vi "RT_Coriolis_Moment_in_DLR_Navigation_Reference_System(SubVI).vi"(0 "Data":dbl[][](array[numeric]), 2 "le (m) in":dbl, 5 "i":i32, 9 "DCM":dbl[][](array[numeric]), 11 "W_b (rad/s) in":dbl[](array[numeric])) -> (4 "Mco (Nm)":dbl[](array[numeric]))   [LabVIEW 2011]
uses:
  <vilib>/Analysis/Matrix/Datatypes/RealMatrix.ctl
  <vilib>/Analysis/Matrix/Numeric/Conversions/Array To Matrix - RA.vi
  <vilib>/Analysis/Matrix/Numeric/Conversions/Array To Matrix - RA2.vi
  <vilib>/Analysis/baseanly.llb/Real A x B.vi
  <vilib>/Analysis/Matrix/Numeric/Conversions/Matrix To Array - RM.vi
  <vilib>/Analysis/NI_AALBase.lvlib
  <vilib>/Analysis/Matrix/NI_Matrix.lvlib
  <vilib>/Analysis/NI_AALPro.lvlib
panel:
  out "-I_p_matrix (kg.m^2/s)":T1
  out "OMEGA":dbl[](array[numeric])
  out "m":dbl
  out "Re":dbl[](array[numeric])
  out "re":dbl
  out "CoG (m)":dbl
  out "M_p (kg/s)":dbl
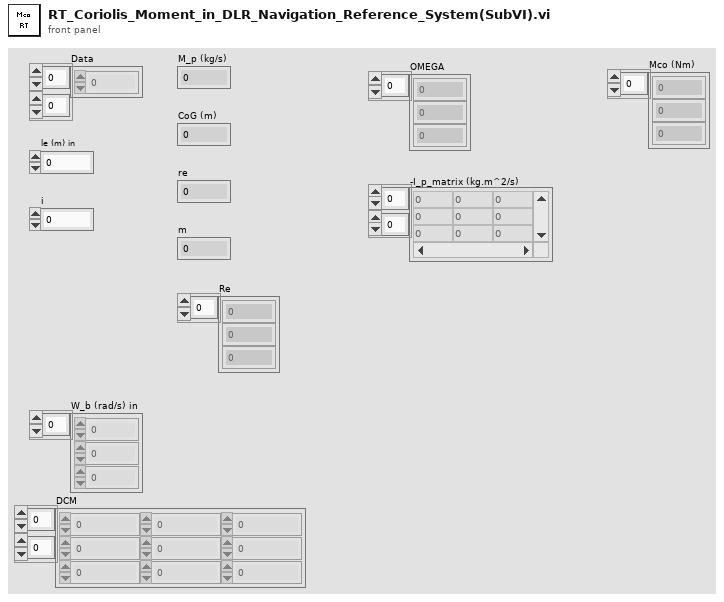
[diagram p1: front panel]
types:
  T1 = typedef "NI_Matrix.lvlib/RealMatrix.ctl" = dbl[][]
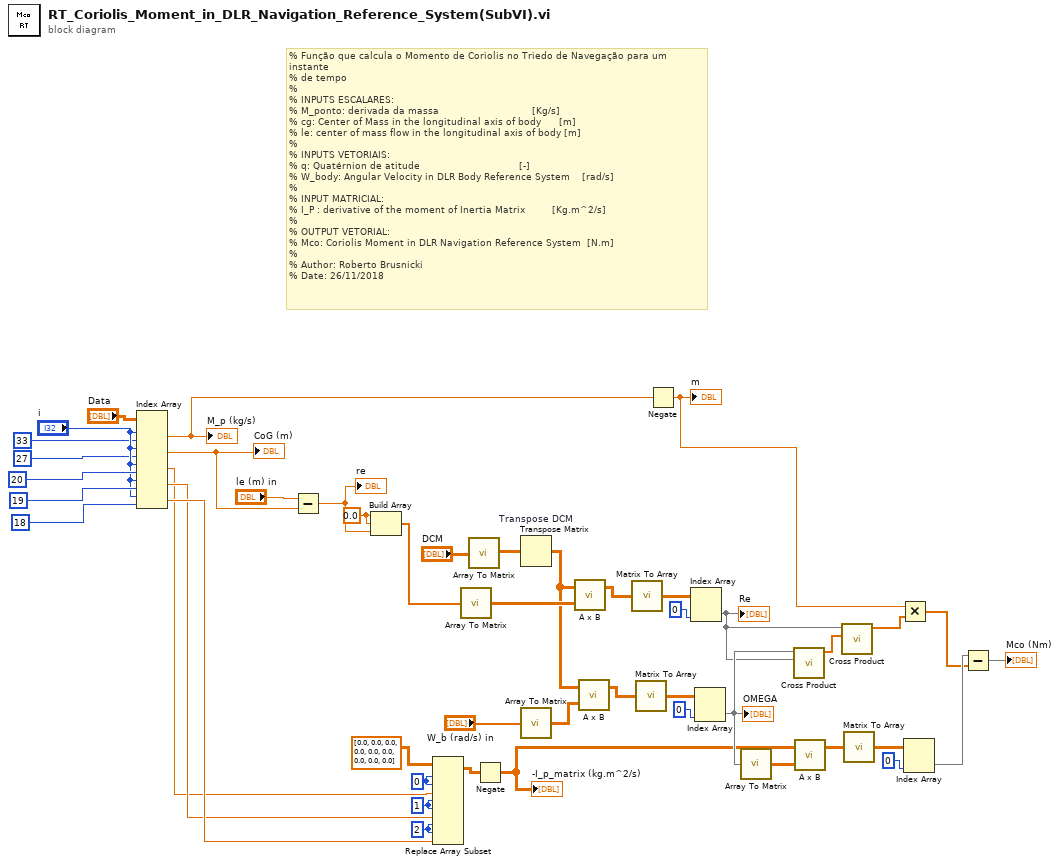
[diagram p0: block diagram]
diagram:
  w32 = 2 ("index (col)")
  w29 = 1 ("index (row)")
  w24 = 0 ("index (col)")
  w12 = 0.0 ("element")
  # "% Função que calcula o Momento de Coriolis no Triedo de Navegação para um instante\n% de tempo\n%\n% INPUTS ESCALARES:\n% M_ponto: derivada da massa                               [Kg/s]\n% cg: Center of Mass in the longitudinal axis of body      [m]\n% le: center of mass flow in the longitudinal axis of body [m]\n% \n% INPUTS VETORIAIS:\n% q: Quatérnion de atitude                                 [-]\n% W_body: Angular Velocity in DLR Body Reference System    [rad/s] \t\n%\n% INPUT MATRICIAL:\n% I_P : derivative of the moment of Inertia Matrix         [Kg.m^2/s]\n%\n% OUTPUT VETORIAL:\n% Mco: Coriolis Moment in DLR Navigation Reference System  [N.m]\n%\n% Author: Roberto Brusnicki\n% Date: 26/11/2018"
  n1 = Index Array(array="Data", index (row) #1="i", index (col) #1=33 ("disabled index (col)"), index (row) #2="i", index (col) #2=27 ("disabled index (col)"), index (row) #3="i", index (col) #3=20 ("disabled index (col)"), index (row) #4="i", index (col) #4=19 ("disabled index (col)"), index (row) #5="i", index (col) #5=18 ("disabled index (col)")) -> (element #1=w9:dbl, element #2=w17:dbl, element #3=w28:dbl, element #4=w30:dbl, element #5=w31:dbl)
  "M_p (kg/s)" <- w9
  "CoG (m)" <- w17
  n2 = Subtract(x="le (m) in", y=w17) -> (x-y=w13:dbl)
  "re" <- w13
  n3 = Build Array(w12, w12, w13) -> (w11:dbl[])
  n4 = Replace Array Subset(array=T1 [[0.0, 0.0, 0.0], [0.0, 0.0, 0.0], [0.0, 0.0, 0.0]] ("transposed matrix"), new element #1=w28, index (row) #1=w24, index (col) #1=w24, new element #2=w30, index (row) #2=w29, index (col) #2=w29, new element #3=w31, index (row) #3=w32, index (col) #3=w32) -> (w34:T1)
  n5 = call-poly <vilib>:"Array To Matrix.vi"("Real 1D Array"=w11) -> ("Real Matrix (Column Vector)"=w14:T1)
  n6 = call-poly <vilib>:"Array To Matrix.vi"("Real 2D Array"="DCM") -> ("Real Matrix"=w10:T1)
  n7 = Negate(x=w34) -> (-x=w35:T1)
  "-I_p_matrix (kg.m^2/s)" <- w35
  n8 = Transpose Matrix "Transpose DCM"(1:w10) -> (0:w6:T1)
  n9 = call-poly <vilib>:"Array To Matrix.vi"("Real 1D Array"="W_b (rad/s) in") -> ("Real Matrix (Column Vector)"=w8:T1)
  n10 = call-poly <vilib>:"A x B.vi"("B"=w14, "A"=w6) -> ("A x B"=w16:T1)  [unwired: 1 out]
  n11 = call-poly <vilib>:"A x B.vi"("B"=w8, "A"=w6) -> ("A x B"=w33:T1)  [unwired: 1 out]
  n12 = call-poly <vilib>:"Matrix To Array.vi"("Real Matrix"=w16) -> ("Real 2D Array"=w15:dbl[][])
  n13 = call-poly <vilib>:"Matrix To Array.vi"("Real Matrix"=w33) -> ("Real 2D Array"=w7:dbl[][])
  n14 = Negate(x=w9) -> (-x=w39:dbl)
  "m" <- w39
  n15 = Index Array(array=w15, index (col)=0 ("index (row)")) -> (element=w36:dbl[])  [unwired: 1 in]
  "Re" <- w36
  n16 = Index Array(array=w7, index (col)=0 ("index (row)")) -> (element=w41:dbl[])  [unwired: 1 in]
  "OMEGA" <- w41
  n17 = call-poly <vilib>:"Array To Matrix.vi"("Real 1D Array"=w41) -> ("Real Matrix (Column Vector)"=w42:T1)
  n18 = call <vilib>:"Cross Product.vi"("B Vector"=w36, "A Vector"=w41) -> ("Cross Product"=w37:dbl[])  [unwired: 8 in, 1 out]
  n19 = call-poly <vilib>:"A x B.vi"("B"=w42, "A"=w35) -> ("A x B"=w40:T1)  [unwired: 1 out]
  n20 = call <vilib>:"Cross Product.vi"("B Vector"=w37, "A Vector"=w36) -> ("Cross Product"=w38:dbl[])  [unwired: 8 in, 1 out]
  n21 = call-poly <vilib>:"Matrix To Array.vi"("Real Matrix"=w40) -> ("Real 2D Array"=w43:dbl[][])
  n22 = Multiply(x=w39, y=w38) -> (x*y=w44:dbl[])
  n23 = Index Array(array=w43, index (col)=0 ("index (row)")) -> (element=w45:dbl[])  [unwired: 1 in]
  n24 = Subtract(x=w45, y=w44) -> (x-y=→"Mco (Nm)":dbl[])
